vi "pmu_Check GPS Information Validity.vi"(7 "unlocked first index":i32, 8 "samples to read":u32, 9 "initial samples to read":u32, 10 "GPS information":T1[](array[typedef]), 11 "reporting GPS information in":T1) -> (3 "reporting GPS information out":T1)   [LabVIEW 2011, in "NI_EP_PMU.lvlib"]
doc: "Force the output to be unlocked when the calculated data contains unlocked data."
uses:
  <vilib>/addons/Electrical Power/PMU/NI_EP_PMU.lvlib
  <vilib>/addons/Electrical Power/PMU/Common/Controls/pmu_GPS Info.ctl
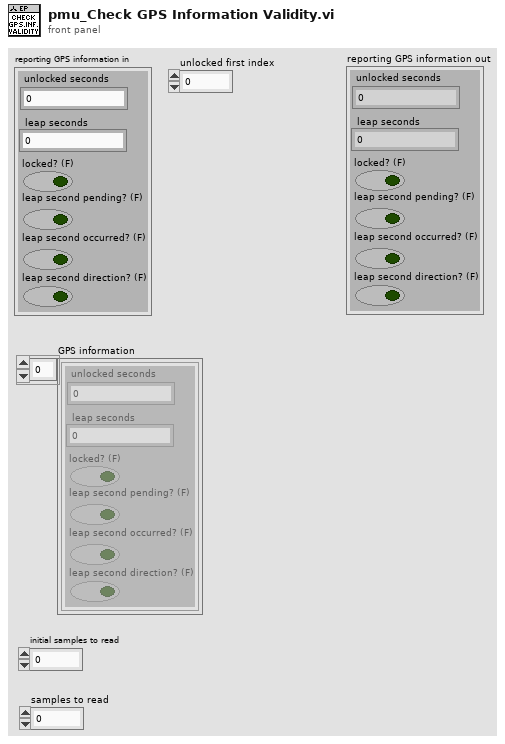
[diagram p1: front panel]
types:
  T1 = typedef "NI_EP_PMU.lvlib/pmu_GPS Info.ctl" = cluster{"unlocked seconds":u32, "leap seconds":i8, "locked? (F)":bool, "leap second pending? (F)":bool, "leap second occurred? (F)":bool, "leap second direction? (F)":bool}
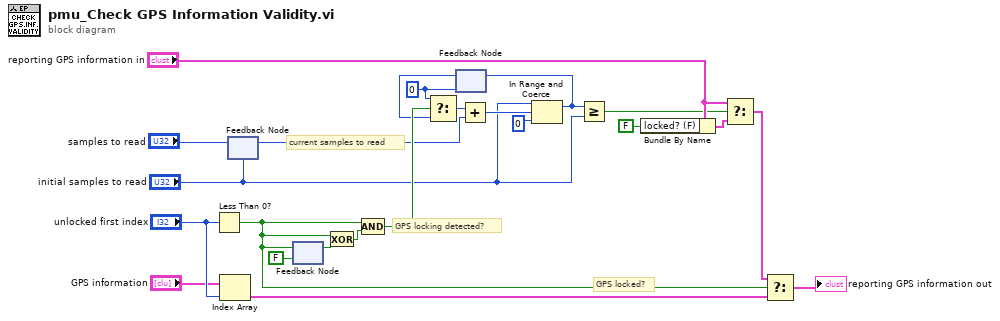
[diagram p0: block diagram]
diagram:
  w23 = u32 0 ("f")
  # "GPS locked?"
  # "current samples to read"
  # "GPS locking detected?"
  n1 = Less Than 0?(x="unlocked first index") -> (x < 0?=w8:bool)
  n2 = Index Array(array="GPS information", index="unlocked first index") -> (element=w5:T1)
  n3 = feedback #1("initial samples to read") -> (w2:u32)
  n4 = feedback-in #1("samples to read") -> ()
  n5 = feedback #2(FALSE) -> (w20:bool)
  n6 = feedback-in #2(w8) -> ()
  n7 = Exclusive Or(1:w20, 2:w8) -> (0:w21:bool)
  n8 = Compound Arithmetic op=AND(w8, w21) -> (w22:bool)
  n9 = feedback #3(w23) -> (w18:u32)
  n10 = Select(t=w23, s=w22, f=w18) -> (s? t:f=w13:u32)
  n11 = Add(x=w13, y=w2) -> (x+y=w12:u32)
  n12 = In Range and Coerce(upper limit="initial samples to read", x=w12, lower limit=u32 0 ("f")) -> (coerced(x)=w10:u32)  [unwired: 1 out]
  n13 = feedback-in #3(w10) -> ()
  n14 = Greater Or Equal?(x=w10, y="initial samples to read") -> (x >= y?=w15:bool)
  n15 = Bundle By Name(cluster="reporting GPS information in", "locked? (F)"=FALSE) -> (w17:T1)
  n16 = Select(t="reporting GPS information in", s=w15, f=w17) -> (s? t:f=w6:T1)
  n17 = Select(t=w6, s=w8, f=w5) -> (s? t:f=→"reporting GPS information out":T1)
